vi "Init.vi"(8 "error in (no error)":errorcluster, 10 "Shutdown Event":refnum<user-event>, 11 "LINX in":refnum<class "LINX.lvclass">) -> (0 "error out":errorcluster, 3 "LINX out":refnum<class "LINX.lvclass">)   [LabVIEW 2019, in "LINX.lvlib" / "LINX.lvclass"]
uses:
  LINX.lvclass
  Plugin Interfaces/Controller Interface/Controller Interface.lvlibp/Controller Interface Class/Controller Interface.lvclass
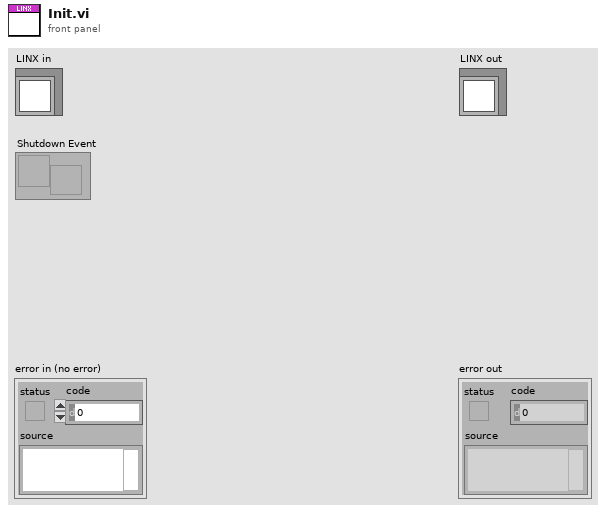
[diagram p1: front panel]
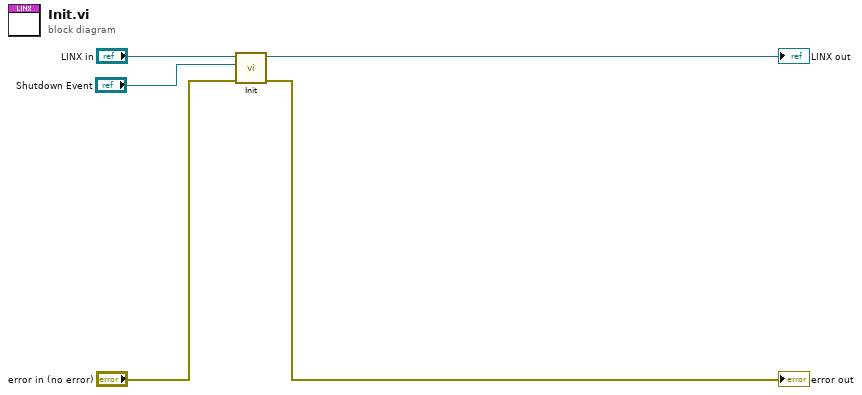
[diagram p0: block diagram]
diagram:
  n1 = call-parent "Init.vi"("error in (no error)"="error in (no error)", "Shutdown Event"="Shutdown Event", "Controller Interface in"="LINX in") -> ("error out"=→"error out":errorcluster, "Controller Interface out"=→"LINX out":refnum<class "LINX.lvclass">)  [unwired: 7 in]
